vi "Common Device Queue Execute Command.vi"(0 "Common Command":string, 11 "VI Refnum":refnum<vi>) -> (4 "Common Command":string, 15 "Quit?":bool)   [LabVIEW 2025]
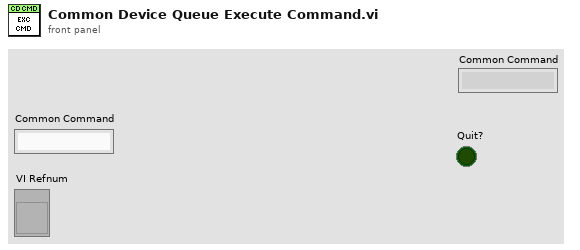
[diagram p1: front panel]
types:
  T1 = enum32{"Invalid", "Standard", "Closed", "Hidden", "Minimized", "Maximized"}
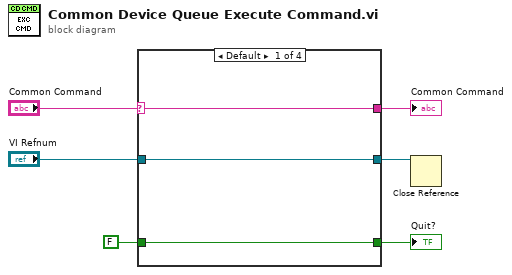
[diagram p0: block diagram]
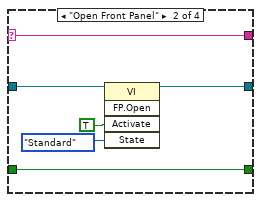
[diagram p2: hidden frame]
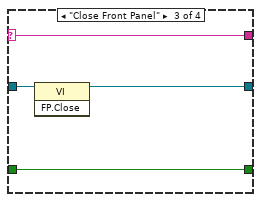
[diagram p3: hidden frame]
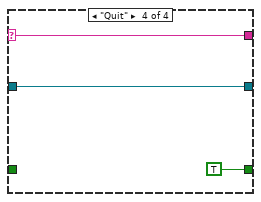
[diagram p4: hidden frame]
diagram:
  n1 = case shown="Default" "Common Command" {
    selector: "Common Command" -> [w7 w10 w16 w20]
    tunnel: "VI Refnum" -> [w8 w13 w19 w21]
    tunnel: [w9 w12 w18 TRUE] -> w4
    tunnel: FALSE -> [w9 w12 w18 _]
    tunnel: [w8 w11 w17 w21] -> w2
    tunnel: [w7 w10 w16 w20] -> w1
    frame Default {
    }
    frame "Open Front Panel" {
      n2 = invoke class="VI" method="FP.Open"(reference=w13, "Activate"=TRUE ("Activate?"), "State"=T1."Standard") -> (reference out=w11:refnum<vi>)  [unwired: 2 in, 4 out]
    }
    frame "Close Front Panel" {
      n3 = invoke class="VI" method="FP.Close"(reference=w19) -> (reference out=w17:refnum<vi>)  [unwired: 2 in, 2 out]
    }
    frame "Quit" {
    }
  }
  "Quit?" <- w4
  "Common Command" <- w1
  n4 = Close Reference(reference=w2) -> ()  [unwired: 1 in, 1 out]
